vi "Reports.Report Config - Dialog.vi"(11 "Report Config":T1[](array[typedef])) -> (1 "OK":bool, 3 "Report Config Out":T1[](array[typedef]))   [LabVIEW 2019]
uses:
  Report.Report File Config Item.ctl
  Report.Report File Type.ctl
panel:
  out "Tab Control":enum32{"Data", "Output"}(tab)
  in  "Cancel Button":bool
  in  "OK Button":bool
  # "Report Setup"
  # "If a sequence name is listed, then the report will be sent to the corresponding folder.\nIf the sequenceis not in the list then the report will be sent to the first folder (the default folder)."
  # "Name/Type"
  # "Sequence                                                                                    Output Folder"
  # "Report Name                                  Sequence Name                                                                                      Output Folder"
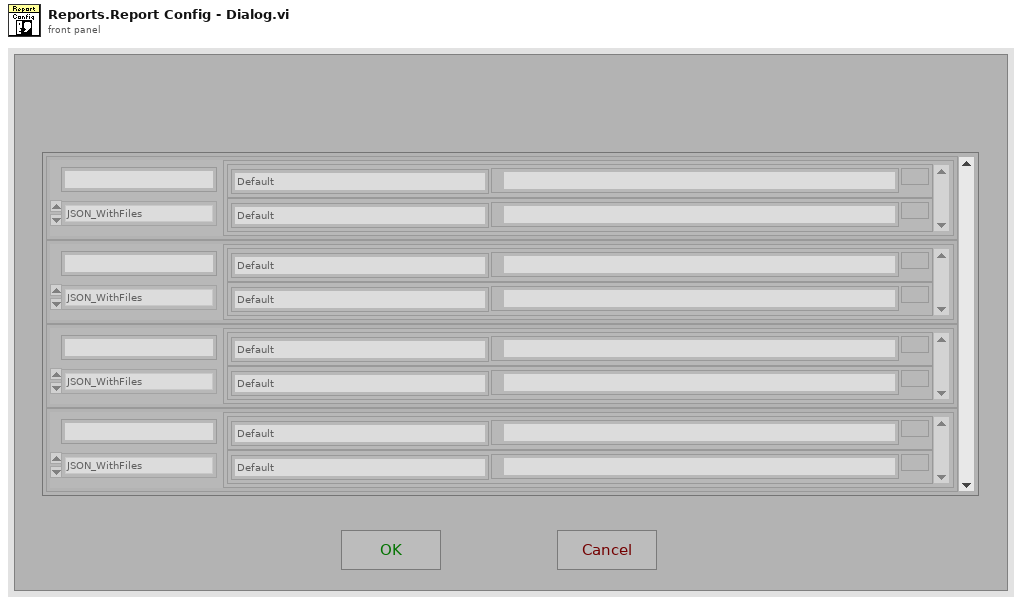
[diagram p1: front panel]
types:
  T1 = typedef "Report.Report File Config Item.ctl" = cluster{"Name":string, "Type":T2, "Seq_Dir":cluster{"Sequence":string, "Folder":path}[]}
  T2 = typedef "Report.Report File Type.ctl" = enum16{"CSV_WithConfigAndData", "CSV", "CSV_SummaryResult", "JSON", "JSON_WithFiles", "XLINK", "XLINK_ResultOnly", "SFC1", ""}
  T3 = enum32{"Invalid", "Standard", "Closed", "Hidden", "Minimized", "Maximized"}
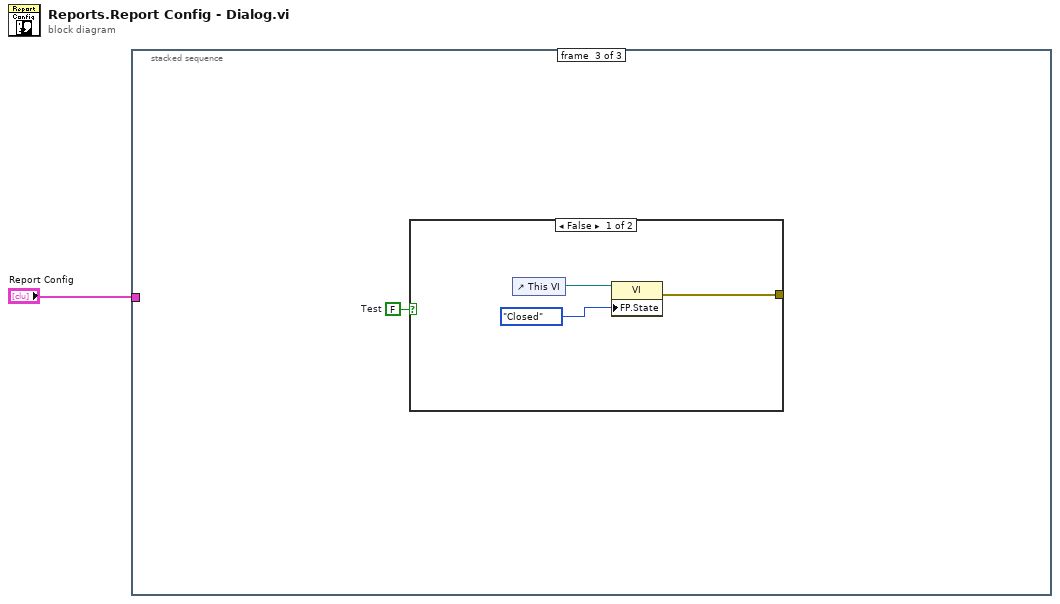
[diagram p0: block diagram]
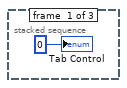
[diagram p2: hidden frame]
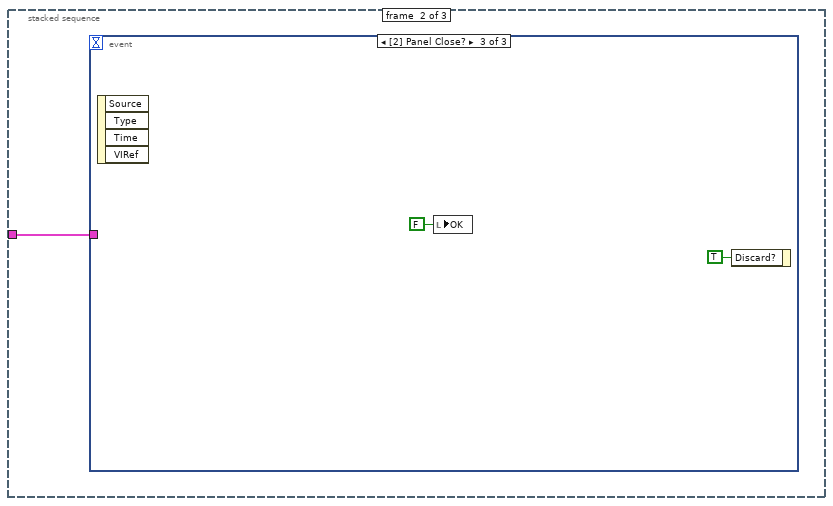
[diagram p3: hidden frame]
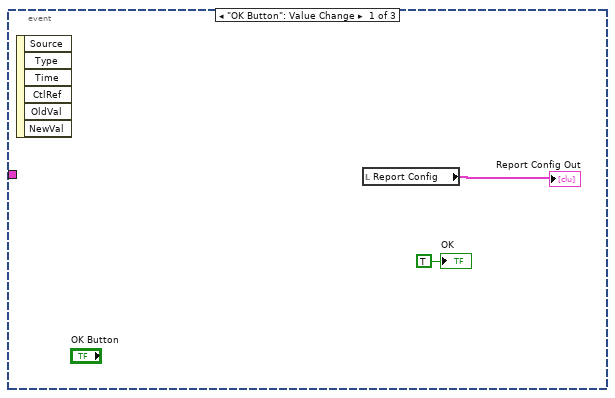
[diagram p4: hidden frame]
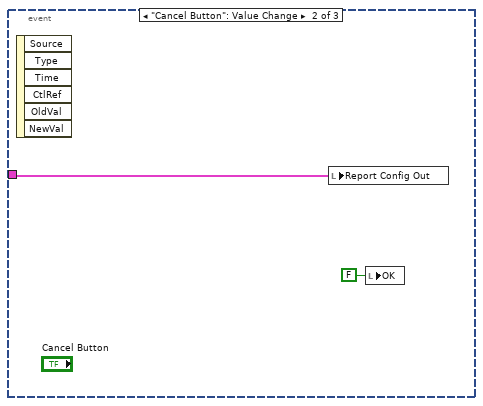
[diagram p5: hidden frame]
diagram:
  n1 = stacked-sequence {
    tunnel: "Report Config" -> [_ w3 _]
    frame #0 {
      "Tab Control" <- 0
    }
    frame #1 {
      n2 = event shown="[2] Panel Close?" {
        selector: _ -> [_ _ _]
        dyn-events: _ -> [_ _ _]
        timeout: _ -> [_ _ _]
        tunnel: w3 -> [_ w6 _]
        event "OK Button": Value Change {
          n3 = event-data() -> ()  [unwired: 1 in, 6 out]
          n4 = local read "Report Config"() -> (→"Report Config Out":T1[])
          "OK" <- TRUE ("OK")
        }
        event "Cancel Button": Value Change {
          n5 = event-data() -> ()  [unwired: 1 in, 6 out]
          n6 = local write "Report Config Out"(w6) -> ()
          n7 = local write "OK"(FALSE ("OK")) -> ()
        }
        event Panel Close? {
          n8 = event-data() -> ()  [unwired: 1 in, 4 out]
          n9 = local write "OK"(FALSE ("OK")) -> ()
          n10 = event-data("Discard?"=TRUE) -> ()  [unwired: 1 in, 1 out]
        }
      }
    }
    frame #2 {
      w10 = FALSE  # Test
      n11 = case shown="False" w10 {
        tunnel: [w11 _] -> _
        frame False {
          n12 = control-ref of="This VI"() -> (w13:refnum<vi>)
          n13 = property class="VI"(reference=w13, "FP.State"=T3."Closed" ("Front Panel Window:State")) -> (error out=w11:errorcluster)  [unwired: 1 in, 1 out]
        }
        frame True {
        }
      }
    }
  }
